vi "Detect Cell Change.vi"(9 "new values":string[][](array[string]), 10 "old values":string[][](array[string])) -> (0 "line removed":bool, 1 "new line":bool, 2 "Cluster":T1, 3 "value change":bool)   [LabVIEW 2013, in "Table Manager.lvlib"]
uses:
  Table Manager.lvlib
  Cell Change.ctl
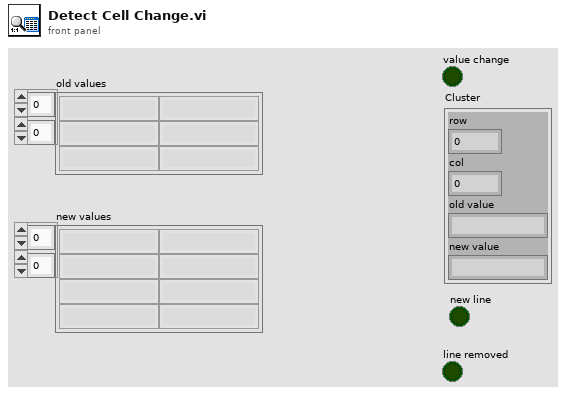
[diagram p1: front panel]
types:
  T1 = typedef "Table Manager.lvlib/Cell Change.ctl" = cluster{"row":i32, "col":i32, "old value":string, "new value":string}
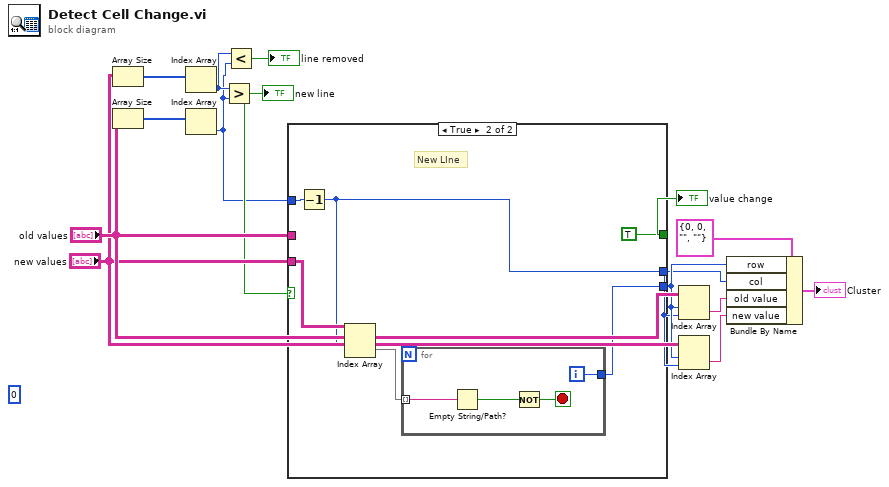
[diagram p0: block diagram]
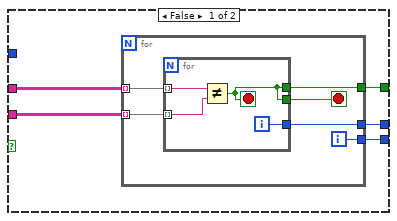
[diagram p2: hidden frame]
diagram:
  (unwired) 0 ("disabled index (col)")
  n1 = Array Size(array="new values") -> (size(s)=w15:i32[])
  n2 = Array Size(array="old values") -> (size(s)=w4:i32[])
  n3 = Index Array(array=w15) -> (element=w3:i32)  [unwired: 1 in]
  n4 = Index Array(array=w4) -> (element=w2:i32)  [unwired: 1 in]
  n5 = Greater?(x=w3, y=w2) -> (0:w5:bool)
  "new line" <- w5
  n6 = Less?(x=w3, y=w2) -> (x < y?=→"line removed":bool)
  n7 = case shown="True" w5 {
    tunnel: [w20 TRUE] -> w14
    tunnel: "old values" -> [w19 _]
    tunnel: "new values" -> [w18 w34]
    tunnel: [w17 w31] -> w7
    tunnel: [w16 w33] -> w6
    tunnel: w2 -> [_ w35]
    frame False {
      n8 = for {
        tunnel: w19 -> [w26] mode=indexing
        tunnel: w18 -> [w25] mode=indexing
        tunnel: [w23] -> w20
        tunnel: [w22] -> w17
        tunnel: [w21] -> w16
        i -> [w22]
        stop <- w24 stop-if-true
        n9 = for {
          tunnel: w25 -> [w30] mode=indexing
          tunnel: w26 -> [w29] mode=indexing
          tunnel: [w28] -> w24
          tunnel: [w28] -> w23
          tunnel: [w27] -> w21
          i -> [w27]
          stop <- w28 stop-if-true
          n10 = Not Equal?(x=w29, y=w30) -> (x != y?=w28:bool)
        }
      }
    }
    frame True {
      # "New LIne"
      n11 = Decrement(x=w35) -> (x-1=w33:i32)
      n12 = Index Array(array=w34, index (row)=w33) -> (element=w32:string[])  [unwired: 1 in]
      n13 = for {
        tunnel: w32 -> [w40] mode=indexing
        tunnel: [w38] -> w31
        i -> [w38]
        stop <- w37 stop-if-true
        n14 = Empty String/Path?(string/path=w40) -> (empty?=w39:bool)
        n15 = Not(x=w39) -> (.not. x?=w37:bool)
      }
    }
  }
  "value change" <- w14
  n16 = Index Array(array="old values", index (row)=w7, index (col)=w6) -> (element=w9:string)
  n17 = Index Array(array="new values", index (row)=w7, index (col)=w6) -> (element=w8:string)
  n18 = Bundle By Name(cluster=T1 {"row"=0, "col"=0, "old value"="", "new value"=""} ("Cluster"), "row"=w7, "col"=w6, "old value"=w9, "new value"=w8) -> (→"Cluster":T1)
